vi "LoadOrWriteBenchConfig.vi"(8 "error in (no error)":errorcluster) -> (0 "error out":errorcluster, 3 "BenchConfig":T1)   [LabVIEW 2013]
uses:
  050 - CONFIG/10 - BenchConfig/BenchConfig.ctl
  050 - CONFIG/00 - ApplicationConfig/Ctrls/EnumFgvConfigCommand.ctl
panel:
  # "A configurer"
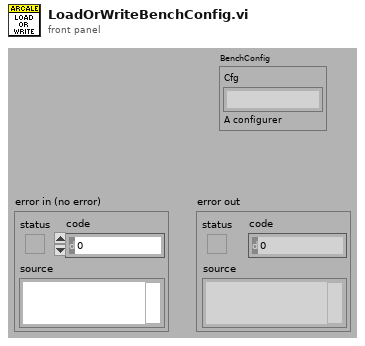
[diagram p1: front panel]
types:
  T1 = typedef "BenchConfig.ctl" = cluster{"Cfg":string}
  T2 = typedef "EnumFgvConfigCommand.ctl" = enum16{"Load", "Get", "Set", "Save To Disk"}
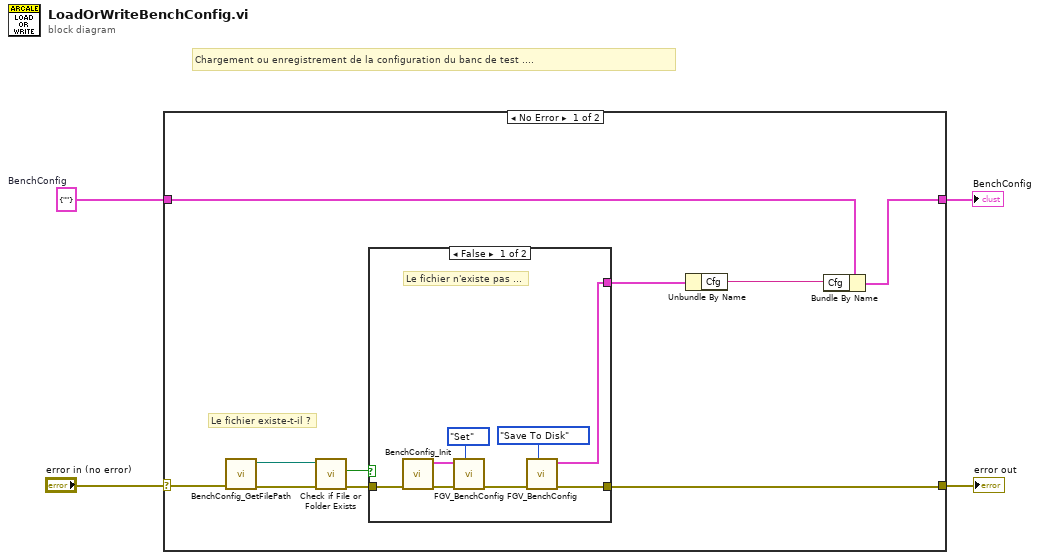
[diagram p0: block diagram]
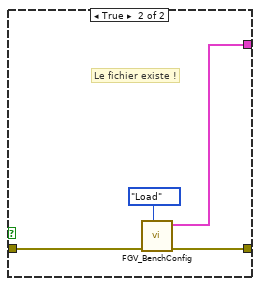
[diagram p2: hidden frame]
diagram:
  w1 = T1 {"Cfg"=""}  # BenchConfig
  # "Chargement ou enregistrement de la configuration du banc de test ...."
  n1 = case shown="No Error" "error in (no error)" {
    selector: "error in (no error)" -> [w14 w28]
    tunnel: [w9 w28] -> w3
    tunnel: w1 -> [w8 w27]
    tunnel: [w7 w27] -> w2
    frame No Error {
      # "Le fichier existe-t-il ?"
      n2 = call "BenchConfig_GetFilePath.vi"("error in (no error)"=w14) -> ("error out"=w13:errorcluster, "BenchConfigFilePath"=w12:path)  [unwired: 9 in]
      n3 = call <vilib>:"Check if File or Folder Exists.vi"("error in (no error)"=w13, "path"=w12) -> ("error out"=w10:errorcluster, "file or folder exists?"=w11:bool)  [unwired: 7 in, 1 out]
      n4 = case shown="False" w11 {
        tunnel: w10 -> [w22 w26]
        tunnel: [w15 w24] -> w6
        tunnel: [w16 w23] -> w9
        frame False {
          # "Le fichier n'existe pas ..."
          n5 = call "BenchConfig_Init.vi"("error in (no error)"=w22) -> ("error out"=w21:errorcluster, "BenchConfig"=w20:T1)  [unwired: 9 in]
          n6 = call "FGV_BenchConfig.vi"("Command"=EnumFgvConfigCommand."Set", "error in (no error)"=w21, "BenchConfigIn"=w20) -> ("error out"=w17:errorcluster)  [unwired: 7 in, 1 out]
          n7 = call "FGV_BenchConfig.vi"("Command"=EnumFgvConfigCommand."Save To Disk", "error in (no error)"=w17) -> ("error out"=w16:errorcluster, "BenchConfigOut"=w15:T1)  [unwired: 8 in]
        }
        frame True {
          # "Le fichier existe !"
          n8 = call "FGV_BenchConfig.vi"("Command"=EnumFgvConfigCommand."Load", "error in (no error)"=w26) -> ("error out"=w23:errorcluster, "BenchConfigOut"=w24:T1)  [unwired: 8 in]
        }
      }
      n9 = Unbundle By Name(w6) -> ("Cfg"=w5:string)
      n10 = Bundle By Name(cluster=w8, "Cfg"=w5) -> (w7:T1)
    }
    frame Error {
    }
  }
  "error out" <- w3
  "BenchConfig" <- w2
